vi "chainManyCommands.vi"(10 "CommandArray":T1, 11 "String in in":string) -> (3 "String out":string)   [LabVIEW 2012]
uses:
  commandArray.ctl
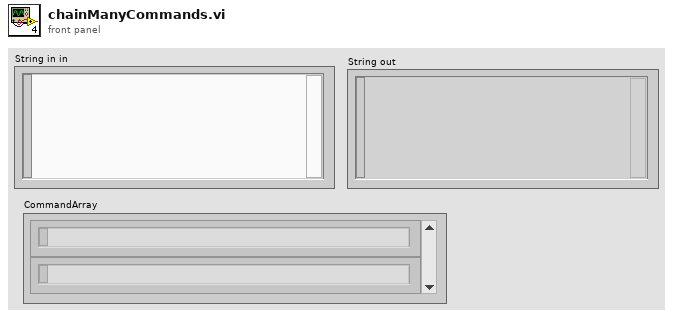
[diagram p1: front panel]
types:
  T1 = typedef "commandArray.ctl" = string[]
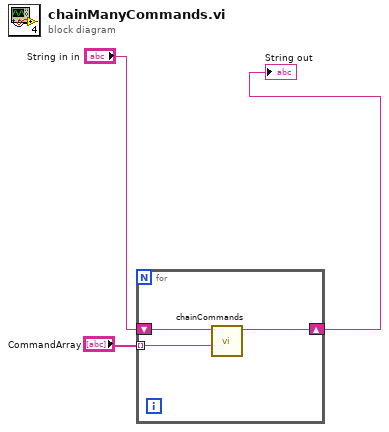
[diagram p0: block diagram]
diagram:
  n1 = for {
    shift-right: [w6] -> w3
    shift-left: "String in in" -> [w5]
    tunnel: "CommandArray" -> [w4] mode=indexing
    n2 = call "chainCommands.vi"("Command"=w4, "StringIn"=w5) -> ("StringOut"=w6:string)  [unwired: 9 in]
  }
  "String out" <- w3
